vi "_Get Mass Ranges.vi"(4 "error in (no error)":errorcluster, 7 "node in":refnum<k20>) -> (0 "error out":errorcluster, 1 "MRParameters":T1[][](array[typedef]), 2 "Mass Ranges":string[][](array[string]), 3 "node out":refnum<k20>)   [LabVIEW 2015]
uses:
  Type/_Mass Range Parameters.ctl
  <vilib>/xml/Close Reference(Node).vi
  <vilib>/xml/NI_XML.lvlib
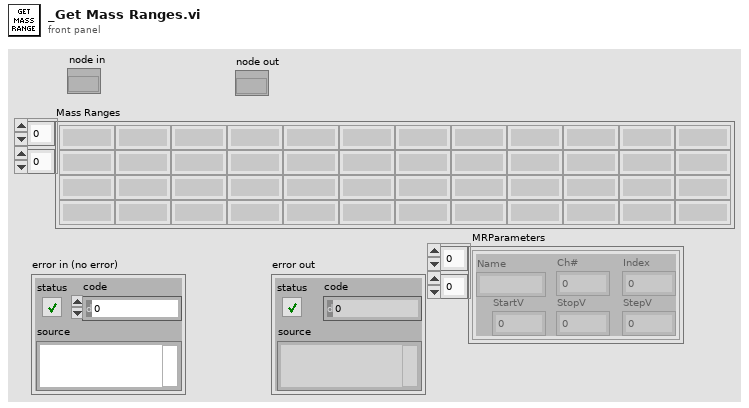
[diagram p1: front panel]
types:
  T1 = typedef "_Mass Range Parameters.ctl" = cluster{"Name":string, "Ch#":u8, "StartV":dbl, "StopV":dbl, "StepV":dbl, "Index":u8}
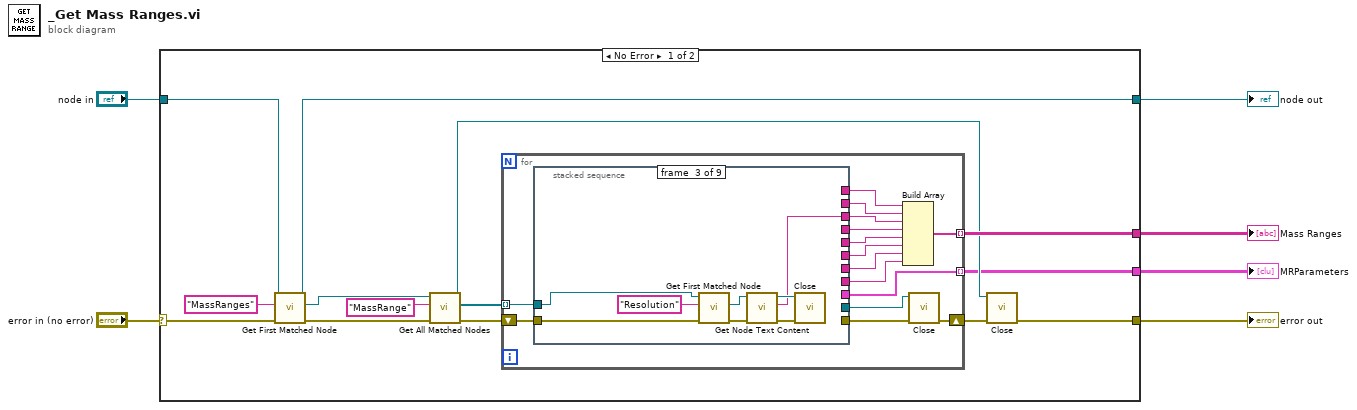
[diagram p0: block diagram]
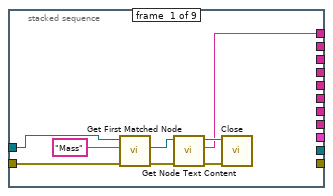
[diagram p2: hidden frame]
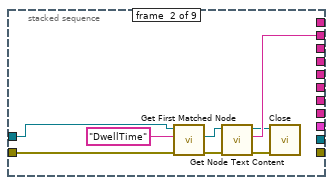
[diagram p3: hidden frame]
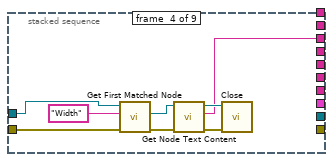
[diagram p4: hidden frame]
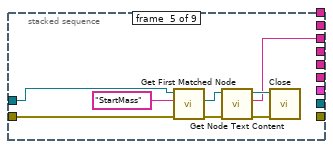
[diagram p5: hidden frame]
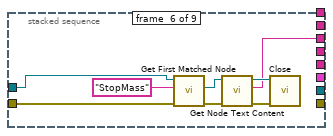
[diagram p6: hidden frame]
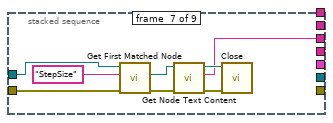
[diagram p7: hidden frame]
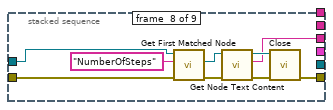
[diagram p8: hidden frame]
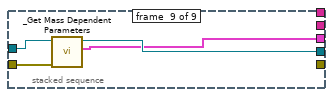
[diagram p9: hidden frame]
diagram:
  n1 = case shown="No Error" "error in (no error)" {
    selector: "error in (no error)" -> [w14 w106]
    tunnel: [w17 _] -> w6
    tunnel: "node in" -> [w15 w105]
    tunnel: [w13 w105] -> w3
    tunnel: [w8 w106] -> w2
    tunnel: [w7 _] -> w1
    frame No Error {
      n2 = call <vilib>:"Get First Matched Node.vi"("error in (no error)"=w14, "XPath expression"="MassRanges", "node in"=w15) -> ("error out"=w11:errorcluster, "node result"=w12:refnum<k20>, "node out"=w13:refnum<k20>)  [unwired: 6 in]
      n3 = call <vilib>:"Get All Matched Nodes.vi"("error in (no error)"=w11, "XPath expression"="MassRange", "node in"=w12) -> ("error out"=w19:errorcluster, "node result array"=w18:refnum<k20>[], "node out"=w9:refnum<k20>)  [unwired: 6 in]
      n4 = for {
        shift-right: [w33] -> w10
        shift-left: w19 -> [w34]
        tunnel: w18 -> [w35] mode=indexing
        tunnel: [w29] -> w17 mode=indexing
        tunnel: [w21] -> w7 mode=indexing
        n5 = stacked-sequence {
          tunnel: w35 -> [w43 w51 w59 w67 w75 w83 w91 w100 w104]
          tunnel: w34 -> [w42 w50 w58 w66 w74 w82 w90 w99 w102]
          tunnel: [w36 _ _ _ _ _ _ _ _] -> w32
          tunnel: [_ w47 _ _ _ _ _ _ _] -> w31
          tunnel: [_ _ w52 _ _ _ _ _ _] -> w30
          tunnel: [_ _ _ _ _ _ _ _ w103] -> w28
          tunnel: [_ _ _ _ _ _ _ w92 _] -> w27
          tunnel: [_ _ _ w60 _ _ _ _ _] -> w26
          tunnel: [_ _ _ _ w68 _ _ _ _] -> w25
          tunnel: [_ _ _ _ _ w76 _ _ _] -> w24
          tunnel: [_ _ _ _ _ _ w84 _ _] -> w23
          tunnel: [_ _ _ _ _ _ _ w93 _] -> w22
          tunnel: [_ _ _ _ _ _ _ _ w101] -> w21
          frame #0 {
            n6 = call <vilib>:"Get First Matched Node.vi"("error in (no error)"=w42, "XPath expression"="Mass", "node in"=w43) -> ("error out"=w39:errorcluster, "node result"=w40:refnum<k20>)  [unwired: 6 in, 1 out]
            n7 = call <vilib>:"Get Node Text Content.vi"("error in (no error)"=w39, "node in"=w40) -> ("error out"=w37:errorcluster, "node text"=w36:string, "node out"=w38:refnum<k20>)  [unwired: 7 in]
            n8 = call-poly <vilib>:"Close.vi"("error in (no error)"=w37, "node"=w38) -> ()  [unwired: 7 in, 1 out]
          }
          frame #1 {
            n9 = call <vilib>:"Get First Matched Node.vi"("error in (no error)"=w50, "XPath expression"="DwellTime", "node in"=w51) -> ("error out"=w44:errorcluster, "node result"=w48:refnum<k20>)  [unwired: 6 in, 1 out]
            n10 = call <vilib>:"Get Node Text Content.vi"("error in (no error)"=w44, "node in"=w48) -> ("error out"=w45:errorcluster, "node text"=w47:string, "node out"=w46:refnum<k20>)  [unwired: 7 in]
            n11 = call-poly <vilib>:"Close.vi"("error in (no error)"=w45, "node"=w46) -> ()  [unwired: 7 in, 1 out]
          }
          frame #2 {
            n12 = call <vilib>:"Get First Matched Node.vi"("error in (no error)"=w58, "XPath expression"="Resolution", "node in"=w59) -> ("error out"=w55:errorcluster, "node result"=w56:refnum<k20>)  [unwired: 6 in, 1 out]
            n13 = call <vilib>:"Get Node Text Content.vi"("error in (no error)"=w55, "node in"=w56) -> ("error out"=w54:errorcluster, "node text"=w52:string, "node out"=w53:refnum<k20>)  [unwired: 7 in]
            n14 = call-poly <vilib>:"Close.vi"("error in (no error)"=w54, "node"=w53) -> ()  [unwired: 7 in, 1 out]
          }
          frame #3 {
            n15 = call <vilib>:"Get First Matched Node.vi"("error in (no error)"=w66, "XPath expression"="Width", "node in"=w67) -> ("error out"=w63:errorcluster, "node result"=w64:refnum<k20>)  [unwired: 6 in, 1 out]
            n16 = call <vilib>:"Get Node Text Content.vi"("error in (no error)"=w63, "node in"=w64) -> ("error out"=w62:errorcluster, "node text"=w60:string, "node out"=w61:refnum<k20>)  [unwired: 7 in]
            n17 = call-poly <vilib>:"Close.vi"("error in (no error)"=w62, "node"=w61) -> ()  [unwired: 7 in, 1 out]
          }
          frame #4 {
            n18 = call <vilib>:"Get First Matched Node.vi"("error in (no error)"=w74, "XPath expression"="StartMass", "node in"=w75) -> ("error out"=w71:errorcluster, "node result"=w72:refnum<k20>)  [unwired: 6 in, 1 out]
            n19 = call <vilib>:"Get Node Text Content.vi"("error in (no error)"=w71, "node in"=w72) -> ("error out"=w70:errorcluster, "node text"=w68:string, "node out"=w69:refnum<k20>)  [unwired: 7 in]
            n20 = call-poly <vilib>:"Close.vi"("error in (no error)"=w70, "node"=w69) -> ()  [unwired: 7 in, 1 out]
          }
          frame #5 {
            n21 = call <vilib>:"Get First Matched Node.vi"("error in (no error)"=w82, "XPath expression"="StopMass", "node in"=w83) -> ("error out"=w79:errorcluster, "node result"=w80:refnum<k20>)  [unwired: 6 in, 1 out]
            n22 = call <vilib>:"Get Node Text Content.vi"("error in (no error)"=w79, "node in"=w80) -> ("error out"=w78:errorcluster, "node text"=w76:string, "node out"=w77:refnum<k20>)  [unwired: 7 in]
            n23 = call-poly <vilib>:"Close.vi"("error in (no error)"=w78, "node"=w77) -> ()  [unwired: 7 in, 1 out]
          }
          frame #6 {
            n24 = call <vilib>:"Get First Matched Node.vi"("error in (no error)"=w90, "XPath expression"="StepSize", "node in"=w91) -> ("error out"=w87:errorcluster, "node result"=w88:refnum<k20>)  [unwired: 6 in, 1 out]
            n25 = call <vilib>:"Get Node Text Content.vi"("error in (no error)"=w87, "node in"=w88) -> ("error out"=w86:errorcluster, "node text"=w84:string, "node out"=w85:refnum<k20>)  [unwired: 7 in]
            n26 = call-poly <vilib>:"Close.vi"("error in (no error)"=w86, "node"=w85) -> ()  [unwired: 7 in, 1 out]
          }
          frame #7 {
            n27 = call <vilib>:"Get First Matched Node.vi"("error in (no error)"=w99, "XPath expression"="NumberOfSteps", "node in"=w100) -> ("error out"=w96:errorcluster, "node result"=w97:refnum<k20>)  [unwired: 6 in, 1 out]
            n28 = call <vilib>:"Get Node Text Content.vi"("error in (no error)"=w96, "node in"=w97) -> ("error out"=w95:errorcluster, "node text"=w93:string, "node out"=w94:refnum<k20>)  [unwired: 7 in]
            n29 = call-poly <vilib>:"Close.vi"("error in (no error)"=w95, "node"=w94) -> ("error out"=w92:errorcluster)  [unwired: 7 in]
          }
          frame #8 {
            n30 = call "_Get Mass Dependent Parameters.vi"("error in (no error)"=w102, "node in"=w104) -> ("Parameters"=w101:T1[], "node out"=w103:refnum<k20>)  [unwired: 3 in, 1 out]
          }
        }
        n31 = Build Array(w32, w31, w30, w26, w25, w24, w23, w22) -> (w29:string[])
        n32 = call-poly <vilib>:"Close.vi"("error in (no error)"=w27, "node"=w28) -> ("error out"=w33:errorcluster)  [unwired: 7 in]
      }
      n33 = call-poly <vilib>:"Close.vi"("error in (no error)"=w10, "node"=w9) -> ("error out"=w8:errorcluster)  [unwired: 7 in]
    }
    frame Error {
    }
  }
  "Mass Ranges" <- w6
  "error out" <- w2
  "node out" <- w3
  "MRParameters" <- w1
